vi "动漫头像生成.vi"() -> ()   [LabVIEW 2021]
panel:
  in  "打开图片文件":bool
  in  "生成头像":bool
  out "new picture":picture caption="生成头像图片"
  in  "设置.pt文件路径":path
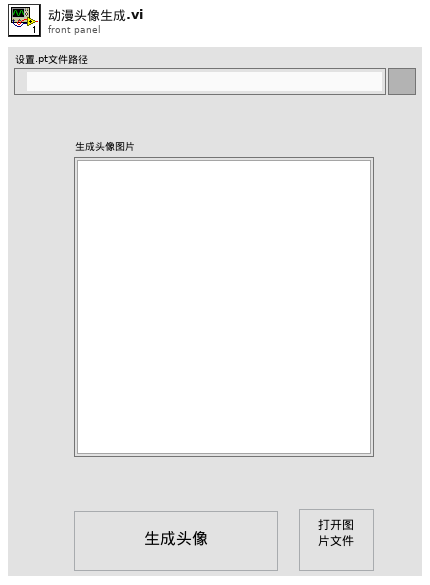
[diagram p1: front panel]
types:
  T1 = typedef "imagedata.ctl" = cluster{"image type":i32, "image depth":i32, "image":u8[], "mask":u8[], "colors":u32[], "Rectangle":cluster{"left":i16, "top":i16, "right":i16, "bottom":i16}}
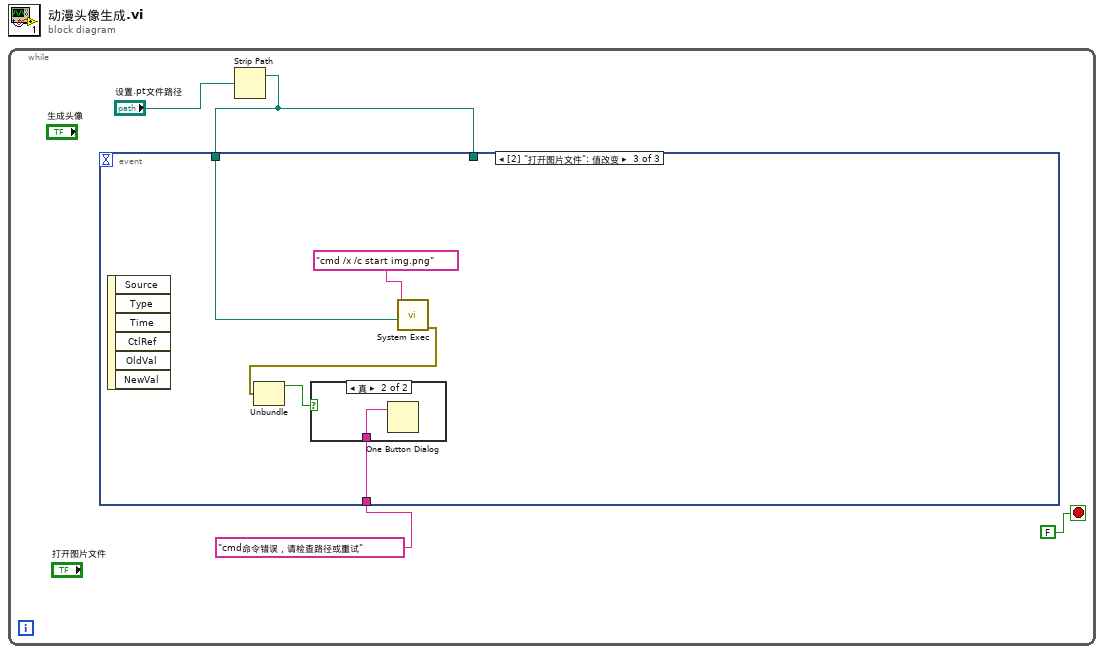
[diagram p0: block diagram]
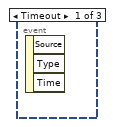
[diagram p2: hidden frame]
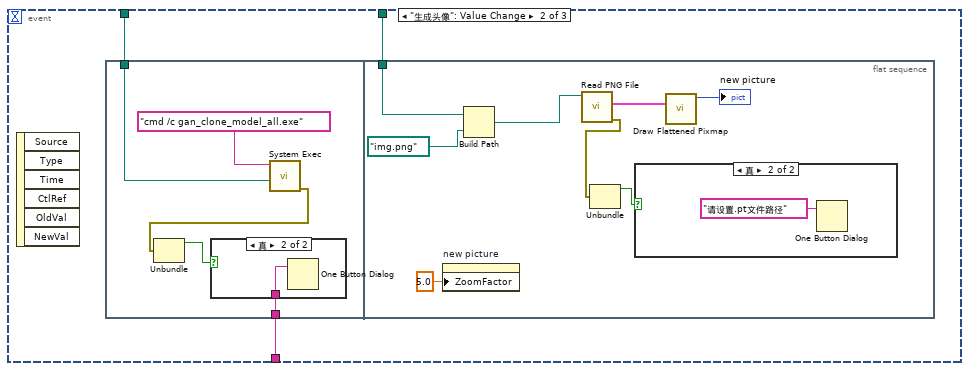
[diagram p3: hidden frame]
diagram:
  n1 = while {
    stop <- FALSE stop-if-true
    n2 = Strip Path(path="设置.pt文件路径") -> (stripped path=w2:path)  [unwired: 1 out]
    n3 = event shown="[2] \"打开图片文件\": 值改变" {
      selector: _ -> [_ _ _]
      dyn-events: _ -> [_ _ _]
      timeout: _ -> [_ _ _]
      tunnel: w2 -> [_ w7 w26]
      tunnel: w2 -> [_ w6 _]
      tunnel: "cmd命令错误，请检查路径或重试" ("消息") -> [_ w5 w23]
      event Timeout {
        n4 = event-data() -> ()  [unwired: 1 in, 3 out]
      }
      event "生成头像": Value Change {
        n5 = event-data() -> ()  [unwired: 1 in, 6 out]
        n6 = flat-sequence {
          tunnel: w7 -> [w12]
          tunnel: w5 -> [w8]
          tunnel: w6 -> [w16]
          frame #0 {
            n7 = call <vilib>:"System Exec.vi"("working directory"=w12, "command line"="cmd /c gan_clone_model_all.exe") -> ("error out"=w10:errorcluster)  [unwired: 6 in, 3 out]
            n8 = Unbundle(w10) -> ("status"=w9:bool)  [unwired: 2 out]
            n9 = case shown="真" w9 {
              tunnel: w8 -> [_ w13]
              frame False {
              }
              frame True {
                n10 = One Button Dialog(message=w13) -> ()  [unwired: 1 in, 1 out]
              }
            }
          }
          frame #1 {
            n11 = property on="new picture" class="Pict"("ZoomFactor"=sgl 5.0 ("缩放因子")) -> ()  [unwired: 2 in, 2 out]
            n12 = Build Path(base path=w16, name or relative path=path "img.png") -> (appended path=w19:path)
            n13 = call <vilib>:"Read PNG File.vi"("path to PNG file"=w19) -> ("error out"=w15:errorcluster, "image data"=w20:T1)  [unwired: 8 in, 1 out]
            n14 = Unbundle(w15) -> ("status"=w14:bool)  [unwired: 2 out]
            n15 = case shown="真" w14 {
              frame False {
              }
              frame True {
                n16 = One Button Dialog(message="请设置.pt文件路径" ("消息")) -> ()  [unwired: 1 in, 1 out]
              }
            }
            n17 = call <vilib>:"Draw Flattened Pixmap.vi"("image data"=w20) -> ("new picture"=→"new picture":picture)  [unwired: 8 in]
          }
        }
      }
      event "打开图片文件": Value Change {
        n18 = event-data() -> ()  [unwired: 1 in, 6 out]
        n19 = call <vilib>:"System Exec.vi"("working directory"=w26, "command line"="cmd /x /c start img.png") -> ("error out"=w24:errorcluster)  [unwired: 6 in, 3 out]
        n20 = Unbundle(w24) -> ("status"=w25:bool)  [unwired: 2 out]
        n21 = case shown="真" w25 {
          tunnel: w23 -> [_ w28]
          frame False {
          }
          frame True {
            n22 = One Button Dialog(message=w28) -> ()  [unwired: 1 in, 1 out]
          }
        }
      }
    }
  }
